vi "main.vi"() -> ()   [LabVIEW 2021]
panel:
  in  "Tab Control":T1(tab)
  in  "?":bool
  out "Files Being Streamed on UDP":string[](array[string])
  in  "UDP Stream On":bool
  in  "Remove File from Stream":bool
  in  "Add File to Stream":bool
  in  "Data Files Available for Streaming":string(combo)
  in  "Data Frequency (Hz)":i32=10
  out "Remaining Data Lines":i32[](array[numeric])
  in  "Skip Points (All Files)":bool
  in  "Number of Points to Skip":i32
  out "Raw Data Array":cluster{string[], i32}[](array[cluster])
  in  "UDP IP Address":string="239.1.4.6"
  in  "UDP Port":u16=50001
  out "System Time":timestamp
  out "error out":errorcluster
  in  "Time-to-live (1)":u16=1
  # "Select a file from the above drop down menu (they must be loaded into the emulator data subdirectory) and click 'Add File' to add the file to those which will be streamed."
  # "Files can be removed from the streamed data by selecting it in the drop down menu and pressing 'Remove File'. Use 'UDP Stream On' to start streaming."
  # "The names of the files being streamed and number of points remaining are displayed on the right. Duplicates of files may not be added to the list of files being streamed."
  # "It is possible to skip points by entering a integer value into 'number of points to skip' and pressing 'Skip Points (All Files)'."
  # "UDP IP Settings"
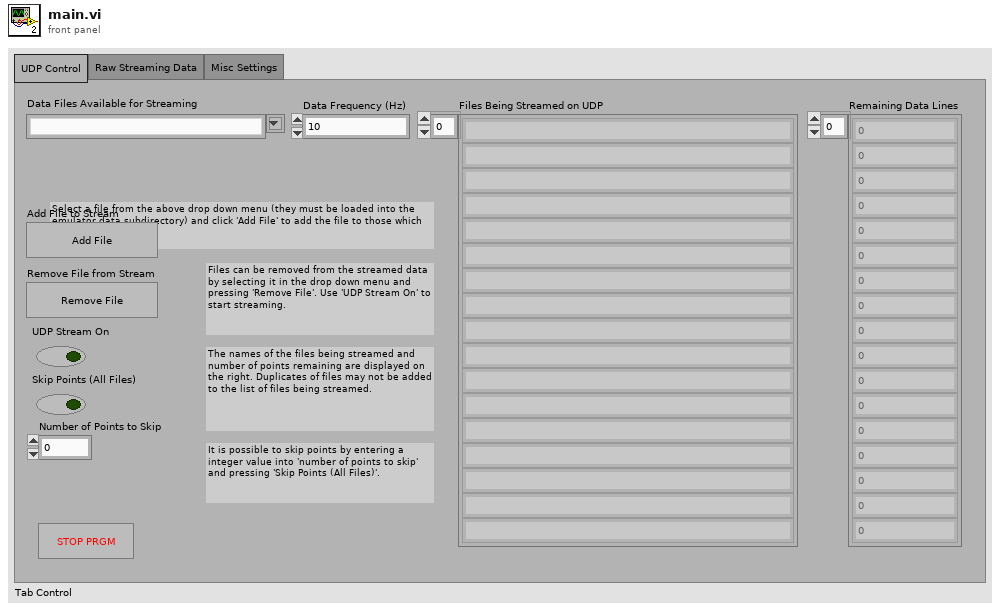
[diagram p1: front panel]
types:
  T1 = enum32{"UDP Control", "Raw Streaming Data", "Misc Settings"}
  T2 = cluster{"Data Array":string[], "Data Frequency (Hz)":i32}
  T3 = cluster{"Data Array":string[], "Data Frequency (Hz)":i32}[]
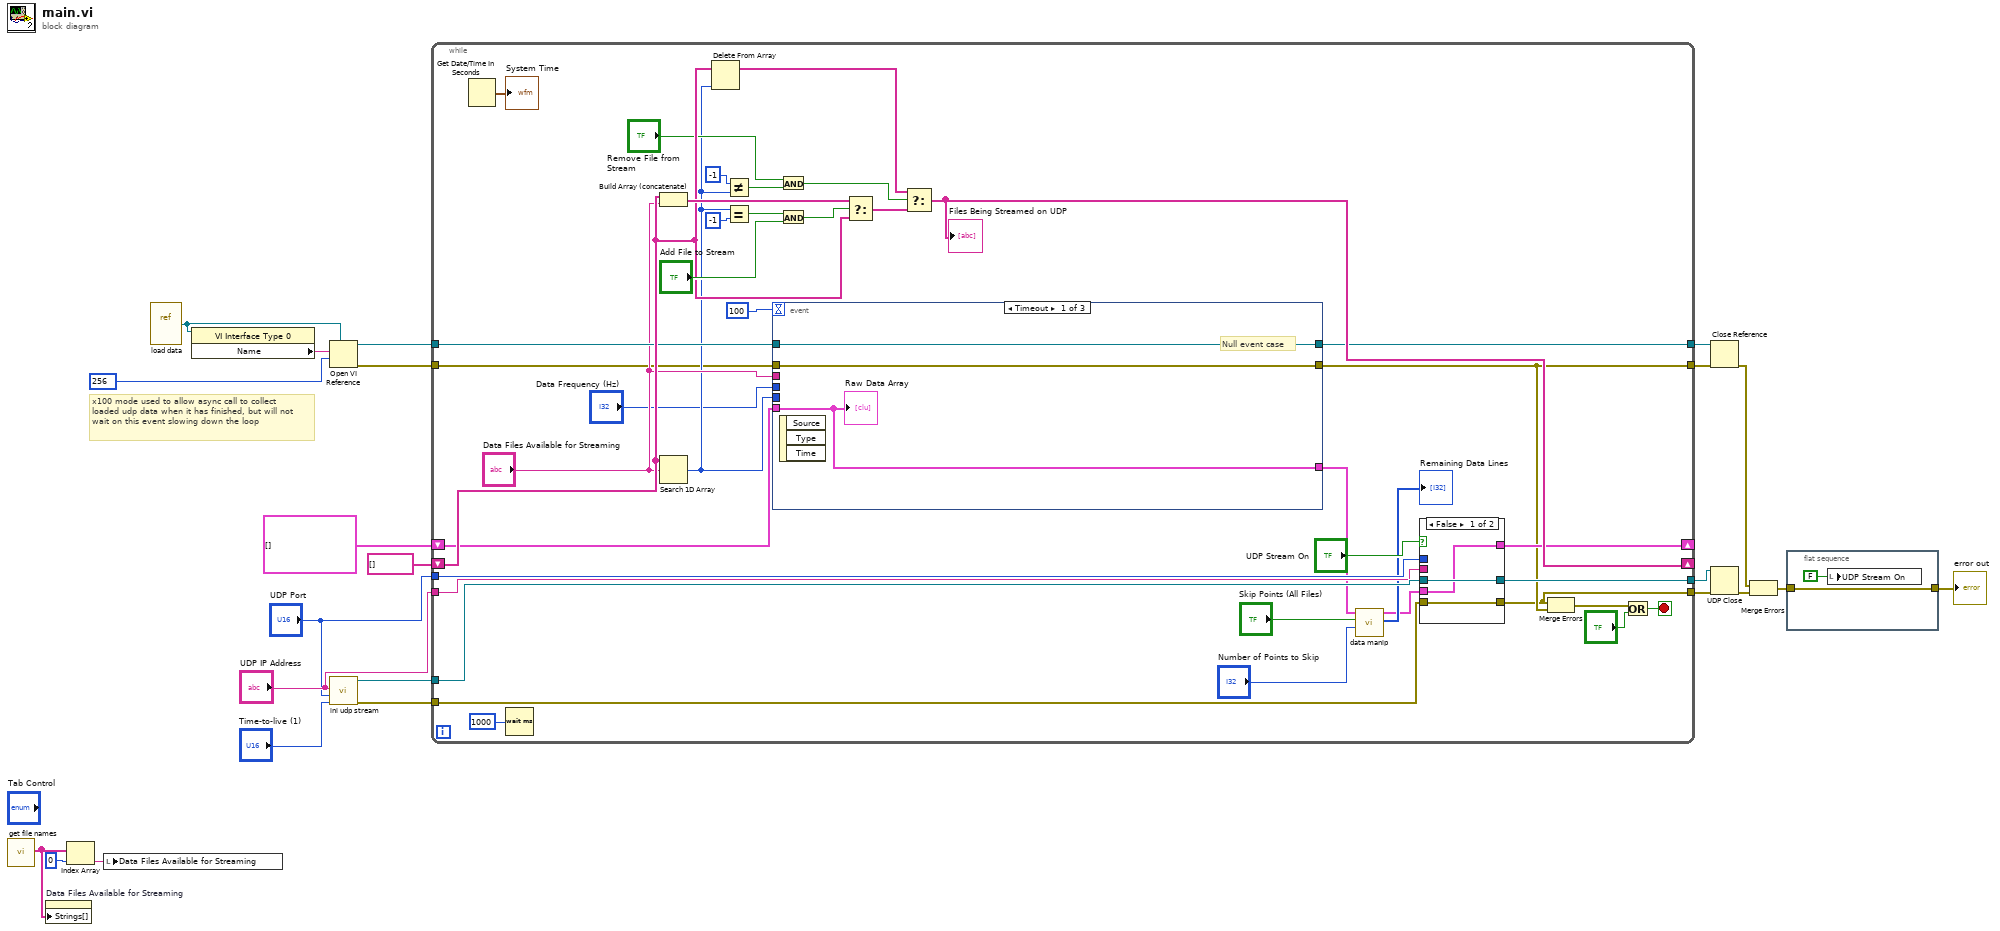
[diagram p0: block diagram]
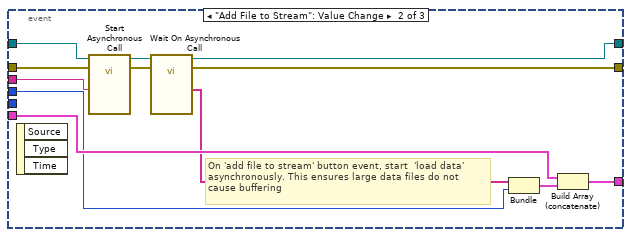
[diagram p2: hidden frame]
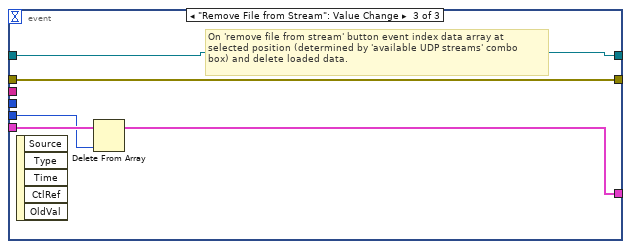
[diagram p3: hidden frame]
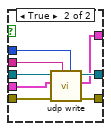
[diagram p4: hidden frame]
diagram:
  # "x100 mode used to allow async call to collect loaded udp data when it has finished, but will not wait on this event slowing down the loop"
  n1 = call "get file names.vi"() -> ("UDP data filenames"=w14:string[])  [unwired: 11 in]
  n2 = property on="Data Files Available for Streaming" class="CmbBox"("Strings[]"=w14) -> ()  [unwired: 2 in, 2 out]
  n3 = Index Array(array=w14, index=0) -> (element=w12:string)
  n4 = local write "Data Files Available for Streaming"(w12) -> ()
  n5 = vi-ref "load data.vi"() -> (w16:refnum<vi>)
  n6 = property class="VI Interface Type 0"(reference=w16) -> ("Name"=w15:string)  [unwired: 1 in, 2 out]
  n7 = Open VI Reference(type specifier VI Refnum (for type only)=w16, vi path=w15, options=256) -> (vi reference=w18:refnum<vi>, error out=w8:errorcluster)  [unwired: 3 in]
  n8 = call "ini udp stream.vi"("time-to-live (default 1)"="Time-to-live (1)", "UDP Port"="UDP Port", "UDP IP Port"="UDP IP Address") -> ("error out udp"=w19:errorcluster, "connection ID"=w22:refnum<k16>)  [unwired: 7 in]
  n9 = while {
    shift-right: [w48] -> _
    shift-left: string[] [] -> [w58]
    tunnel: w22 -> [w52]
    tunnel: [w51] -> w21
    tunnel: [w33] -> w20
    tunnel: w19 -> [w50]
    tunnel: w18 -> [w46]
    tunnel: [w44] -> w11
    tunnel: [w36] -> w10
    shift-right: [w40] -> _
    shift-left: cluster{string[], i32}[] [] -> [w43]
    tunnel: w8 -> [w35]
    tunnel: "UDP IP Address" -> [w32]
    tunnel: "UDP Port" -> [w31]
    stop <- w37 stop-if-true
    n10 = Get Date/Time In Seconds() -> (seconds since 1Jan1904=→"System Time":timestamp)
    n11 = Wait (ms)(milliseconds to wait=u32 1000) -> ()  [unwired: 1 out]
    n12 = Build Array (concatenate)(w58, "Data Files Available for Streaming") -> (w63:string[])
    n13 = Search 1D Array(1D array=w58, element="Data Files Available for Streaming") -> (index of element=w42:i32)  [unwired: 1 in]
    n14 = Delete From Array(array=w58, index=w42) -> (array with subset deleted=w57:string[])  [unwired: 1 in, 1 out]
    n15 = Not Equal?(x=-1, y=w42) -> (x != y?=w53:bool)
    n16 = Equal?(x=w42, y=-1) -> (x = y?=w59:bool)
    n17 = event shown="[0] Timeout" {
      selector: _ -> [_ _ _]
      dyn-events: _ -> [_ _ _]
      timeout: 100 -> [_ _ _]
      tunnel: w46 -> [w66 w77 w79]
      tunnel: "Data Files Available for Streaming" -> [_ w76 _]
      tunnel: [w66 w74 w79] -> w44
      tunnel: [w64 w73 w80] -> w36
      tunnel: w43 -> [w65 w72 w83]
      tunnel: [w65 w69 w81] -> w27
      tunnel: w42 -> [_ _ w82]
      tunnel: w35 -> [w64 w68 w80]
      tunnel: "Data Frequency (Hz)" -> [_ w67 _]
      event Timeout {
        # "Null event case"
        n18 = event-data() -> ()  [unwired: 1 in, 3 out]
        "Raw Data Array" <- w65
      }
      event "Add File to Stream": Value Change {
        # "On 'add file to stream' button event, start  'load data' \nasynchronously. This ensures large data files do not \ncause buffering"
        n19 = event-data() -> ()  [unwired: 1 in, 3 out]
        n20 = call-by-ref "Start Asynchronous Call"(reference=w77, error in=w68, "file name"=w76) -> (reference out=w78:refnum<vi>, error out=w75:errorcluster)  [unwired: 9 in, 2 out]
        n21 = call-by-ref "Wait On Asynchronous Call"(reference=w78, error in=w75) -> (reference out=w74:refnum<vi>, error out=w73:errorcluster, "Data Array"=w70:string[])  [unwired: 10 in, 1 out]
        n22 = Bundle("Data Array"=w70, "Data Frequency (Hz)"=w67) -> (w71:T2)  [unwired: 1 in]
        n23 = Build Array (concatenate)(w72, w71) -> (w69:T3)
      }
      event "Remove File from Stream": Value Change {
        # "On 'remove file from stream' button event index data array at\nselected position (determined by 'available UDP streams' combo\nbox) and delete loaded data."
        n24 = event-data() -> ()  [unwired: 1 in, 5 out]
        n25 = Delete From Array(array=w83, index=w82) -> (array with subset deleted=w81:cluster{string[], i32}[])  [unwired: 1 in, 1 out]
      }
    }
    n26 = And(x="Remove File from Stream", y=w53) -> (x .and. y?=w47:bool)
    n27 = And(x=w59, y="Add File to Stream") -> (x .and. y?=w61:bool)
    n28 = Select(t=w63, s=w61, f=w58) -> (s? t:f=w56:string[])
    n29 = Select(t=w57, s=w47, f=w56) -> (s? t:f=w48:string[])
    "Files Being Streamed on UDP" <- w48
    n30 = call "data manip.vi"("Points to be deleted"="Number of Points to Skip", "Skip points"="Skip Points (All Files)", "UDP Data Array (in)"=w27) -> ("points num array"=→"Remaining Data Lines":i32[], "UDP Data Array (Out)"=w26:cluster{"Array":string[], "Numeric":i32}[])  [unwired: 7 in]
    n31 = case shown="False" "UDP Stream On" {
      tunnel: w52 -> [w86 w94]
      tunnel: [w86 w93] -> w51
      tunnel: [w85 w92] -> w33
      tunnel: w50 -> [w85 w91]
      tunnel: w26 -> [w84 w90]
      tunnel: [w84 w89] -> w40
      tunnel: w32 -> [_ w88]
      tunnel: w31 -> [_ w87]
      frame False {
      }
      frame True {
        n32 = call "udp write.vi"("UDP Port"=w87, "UDP IP Address"=w88, "error in (no error)"=w91, "Data Array of Clusters (in)"=w90, "UDP ID (in)"=w94) -> ("error out"=w92:errorcluster, "Data Array of Cluster (out)"=w89:cluster{"Data Array":string[], "Numeric":i32}[], "UDP ID (out)"=w93:refnum<k16>)  [unwired: 4 in]
      }
    }
    n33 = Merge Errors(w33, w36) -> (w34:errorcluster)
    n34 = Or(x=w34, y="?") -> (x .or. y?=w37:bool)
  }
  n35 = Close Reference(reference=w11, error in (no error)=w10) -> (error out=w5:errorcluster)
  n36 = UDP Close(connection ID=w21, 8:w20) -> (error out=w4:errorcluster)  [unwired: 1 out]
  n37 = Merge Errors(w5, w4) -> (w2:errorcluster)
  n38 = flat-sequence {
    tunnel: [w96] -> w3
    tunnel: w2 -> [w96]
    frame #0 {
      n39 = local write "UDP Stream On"(FALSE ("UDP Stream On")) -> ()
    }
  }
  "error out" <- w3
